vi "Single Value Interpolation.vi"(7 "x":dbl, 8 "Lower Value":dbl, 9 "Lower Position":dbl, 10 "Upper Value":dbl, 11 "Upper Position":dbl) -> (3 "Interpolated Value":dbl)   [LabVIEW 2020, in "Profile Interpolation Engine.lvlib"]
doc: "This VI interpolates a value from a Setpoint given a pair of other point/value combinations."
uses:
  Profile Interpolation Engine.lvlib
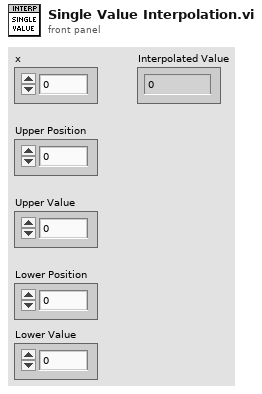
[diagram p1: front panel]
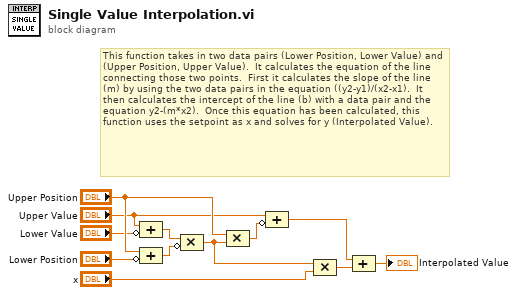
[diagram p0: block diagram]
diagram:
  # "This function takes in two data pairs (Lower Position, Lower Value) and (Upper Position, Upper Value).  It calculates the equation of the line connecting those two points.  First it calculates the slope of the line (m) by using the two data pairs in the equation ((y2-y1)/(x2-x1).  It then calculates the intercept of the line (b) with a data pair and the equation y2-(m*x2).  Once this equation has been calculated, this function uses the setpoint as x and solves for y (Interpolated Value)."
  n1 = Compound Arithmetic op=ADD("Upper Value", invert "Lower Value") -> (w3:dbl)
  n2 = Compound Arithmetic op=ADD("Upper Position", invert "Lower Position") -> (w4:dbl)
  n3 = Compound Arithmetic op=MULTIPLY(w3, invert w4) -> (w9:dbl)
  n4 = Compound Arithmetic op=MULTIPLY("Upper Position", w9) -> (w5:dbl)
  n5 = Compound Arithmetic op=ADD("Upper Value", invert w5) -> (w11:dbl)
  n6 = Compound Arithmetic op=MULTIPLY(w9, "x") -> (w8:dbl)
  n7 = Compound Arithmetic op=ADD(w11, w8) -> (→"Interpolated Value":dbl)
